vi "Move Servo_6.vi"(0 "NXT":T3={"Hardware"="NXT", "Flattened String"=""}, 2 "Servo Position 1":u8=10, 3 "Servo Position 2":u8=10, 4 "Servo Position 3":u8=10, 5 "Servo Position 4":u8=10, 6 "Servo Position 5":u8=10, 7 "Servo Position 6":u8=10, 12 "Servo":T2={"Servo"=enum."Servo", "Address"=-1, "Address"=-1, "Address"=-1, "Address"=-1, "Address"=-1, "Address"=-1}, 14 "Sync (None)":u8(ring) items=["No Sync"=0, "Slow (15)"=15, "Medium (8)"=8, "Fast (1)"=1]) -> (20 "NXT":T3={"Hardware"="NXT", "Flattened String"=""})   [LabVIEW 2010, in "4134Outputs.lvlib"]
uses:
  4134Outputs.lvlib
  <vilib>/NXT/Subs/LVHSConnector.ctl
  <vilib>/NXT/Subs/MotorXNode.Servo Type.ctl
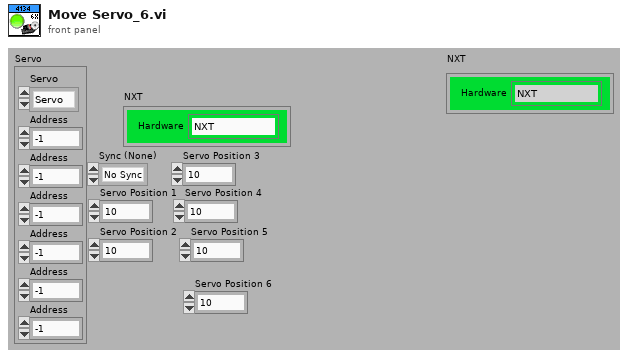
[diagram p1: front panel]
types:
  T1 = typedef "MotorXNode.Servo Type.ctl" = enum16{"Servo"}
  T2 = cluster{"Servo":T1, "Address":i16, "Address":i16, "Address":i16, "Address":i16, "Address":i16, "Address":i16}
  T3 = typedef "LVHSConnector.ctl" = cluster{"Hardware":string, "Flattened String":string}
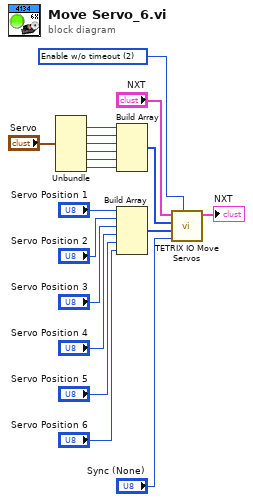
[diagram p0: block diagram]
diagram:
  w19 = u16 2 items=["Disable", "Enable w/timeout", "Enable w/o timeout"] ("Servo State (Enable w/o timeout)")
  n1 = Unbundle("Servo") -> ("Address"=w16:i16, "Address"=w15:i16, "Address"=w14:i16, "Address"=w13:i16, "Address"=w12:i16, "Address"=w11:i16)  [unwired: 1 out]
  n2 = Build Array(w16, w15, w14, w13, w12, w11) -> (w10:i16[])
  n3 = Build Array("Servo Position 1", "Servo Position 2", "Servo Position 3", "Servo Position 4", "Servo Position 5", "Servo Position 6") -> (w9:u8[])
  n4 = call <vilib>:"TETRIX IO Move Servos.vi"("Servo State (Enable w/o timeout)"=w19, "Update Interval (0)"="Sync (None)", "Servo Positions"=w9, "Servos"=w10, "NXT"="NXT") -> ("NXT"=→"NXT":T3)  [unwired: 6 in]
